vi "Refresh.vi"(8 "error in":errorcluster, 11 "SourceGrid in":refnum<class "SourceGrid.lvclass">) -> (0 "error out":errorcluster, 3 "SourceGrid out":refnum<class "SourceGrid.lvclass">)   [LabVIEW 2024, in "SourceGrid.lvlib" / "SourceGrid.lvclass"]
uses:
  SourceGrid.lvclass
  SourceGrid.lvclass/SourceGrid.ctl
  D:/git/Sourcegrid-LabVIEW/dll/SourceGrid.dll
  dll/SourceGrid.dll
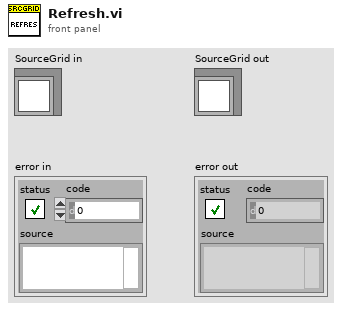
[diagram p1: front panel]
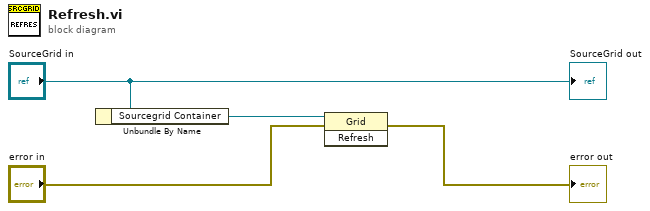
[diagram p0: block diagram]
diagram:
  n1 = Unbundle By Name("SourceGrid in") -> ("Sourcegrid Container"=w3:refnum<k24>)
  n2 = invoke class="Grid" method="Refresh"(reference=w3, error in="error in") -> (error out=→"error out":errorcluster)  [unwired: 1 in, 2 out]
  "SourceGrid out" <- "SourceGrid in"
